vi "Mechanical actions and Structures.vi"() -> ()   [LabVIEW 2020]
panel:
  out "String 5":string
  out "String 4":string
  out "String 3":string
  in  "clc":bool
  in  "/":bool
  in  "*":bool
  in  "-":bool
  in  "+":bool
  out "Boolean 5":bool
  out "Boolean 4":bool
  in  "Enum 2":enum16{"two", "on", "off"}(ring)
  out "Boolean 3":bool
  out "String 2":string
  in  "String":string
  out "Boolean 2":bool
  in  "Boolean":bool
  in  "stop":bool
  out "Array":dbl[](array[numeric])
  out "index":i32
  in  "y":dbl
  in  "x":dbl
  # "case structure by boolen"
  # "case structure by sring"
  # "case structure by enum"
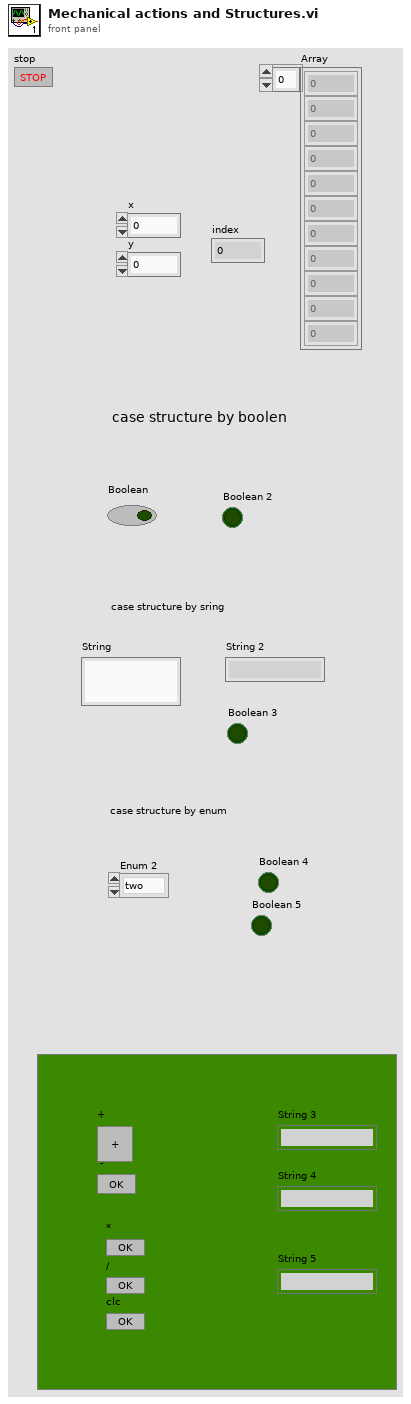
[diagram p1: front panel]
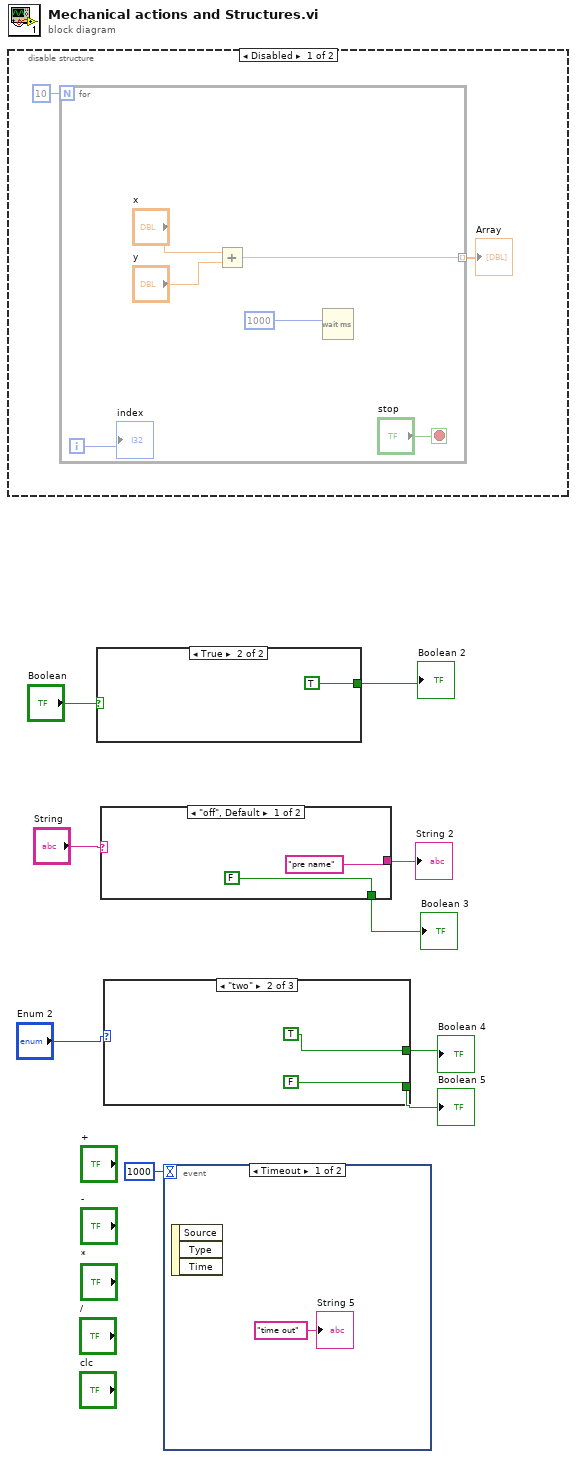
[diagram p0: block diagram]
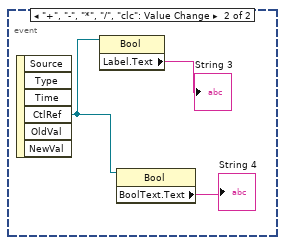
[diagram p2: hidden frame]
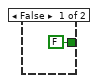
[diagram p3: hidden frame]
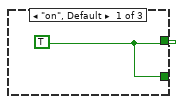
[diagram p4: hidden frame]
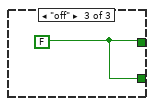
[diagram p5: hidden frame]
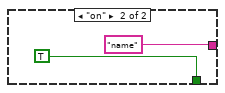
[diagram p6: hidden frame]
diagram:
  n1 = disable-structure shown="Disabled" {
    frame Disabled {
      n2 = for {
        N: 10 -> [_]
        tunnel: [w14] -> w10 mode=indexing
        i -> [w15]
        stop <- "stop" stop-if-true
        n3 = Add(x="x", y="y") -> (x+y=w14:dbl)
        n4 = Wait (ms)(milliseconds to wait=u32 1000 ("millisecond timer value")) -> ()  [unwired: 1 out]
        "index" <- w15
      }
      "Array" <- w10
    }
    frame Enabled {
    }
  }
  n5 = case shown="True" "Boolean" {
    tunnel: [FALSE ("Boolean 2") TRUE ("Boolean 2")] -> w2
    frame False {
    }
    frame True {
    }
  }
  "Boolean 2" <- w2
  n6 = case shown="\"off\", Default" "String" {
    tunnel: ["pre name" "name"] -> w8
    tunnel: [FALSE ("Boolean 2") TRUE ("Boolean 2")] -> w7
    frame "off", Default {
    }
    frame "on" {
    }
  }
  "String 2" <- w8
  "Boolean 3" <- w7
  n7 = case shown="\"two\"" "Enum 2" {
    tunnel: [w24 TRUE w27] -> w5
    tunnel: [w24 FALSE w27] -> w4
    frame "on", Default {
      w24 = TRUE
    }
    frame "two" {
    }
    frame "off" {
      w27 = FALSE
    }
  }
  "Boolean 4" <- w5
  "Boolean 5" <- w4
  n8 = event shown="[0] Timeout" {
    selector: _ -> [_ _]
    dyn-events: _ -> [_ _]
    timeout: 1000 -> [_ _]
    event Timeout {
      n9 = event-data() -> ()  [unwired: 1 in, 3 out]
      "String 5" <- "time out" ("String 5")
    }
    event "+", "-", "*", "/", "clc": Value Change {
      n10 = event-data() -> ("CtlRef"=w30:refnum<vi>)  [unwired: 1 in, 5 out]
      n11 = property class="Bool"(reference=w30) -> ("Label.Text"=→"String 3":string)  [unwired: 1 in, 2 out]
      n12 = property class="Bool"(reference=w30) -> ("BoolText.Text"=→"String 4":string)  [unwired: 1 in, 2 out]
    }
  }
